vi "SRlockin_aux_set.vi"(2 "error in (no error)":errorcluster, 3 "Set Voltage (V)":dbl min=-10.0 max=10.0 step=0.001, 4 "DAC channel":u16=1 min=1 max=4 step=1, 5 "VISA resource name":refnum<visa-resource-name>="GPIB0::8::INSTR") -> (0 "error out":errorcluster, 1 "VISA resource name out":refnum<visa-resource-name>)   [LabVIEW 2018]
panel:
  # "Input parameters"
  # "Output parameters"
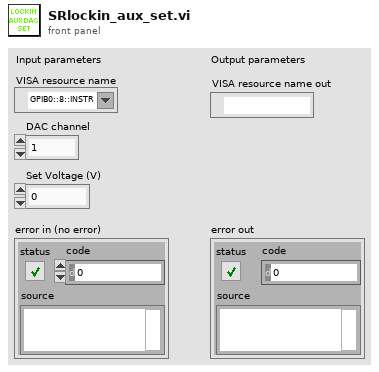
[diagram p1: front panel]
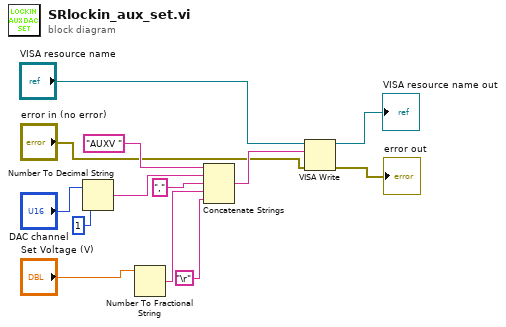
[diagram p0: block diagram]
diagram:
  n1 = Number To Decimal String(number="DAC channel", width (-)=1) -> (decimal integer string=w7:string)
  n2 = Number To Fractional String(number="Set Voltage (V)") -> (F-format string=w5:string)  [unwired: 3 in]
  n3 = Concatenate Strings("AUXV ", w7, ",", w5, "\r") -> (w10:string)
  n4 = VISA Write(VISA resource name="VISA resource name", write buffer=w10, error in (no error)="error in (no error)") -> (VISA resource name out=→"VISA resource name out":refnum<visa-resource-name>, error out=→"error out":errorcluster)  [unwired: 1 out]
